vi "GetName.vi"(8 "error in (no error)":errorcluster, 11 "Konvolucio MCAN120803 Adapter Class in":refnum<class "Konvolucio MCAN120803 Adapter Class.lvclass">) -> (0 "error out":errorcluster, 2 "Value":string, 3 "Konvolucio MCAN120803 Adapter Class out":refnum<class "Konvolucio MCAN120803 Adapter Class.lvclass">)   [LabVIEW 2011, in "Konvolucio MCAN120803 Adapter Class.lvclass"]
uses:
  Konvolucio MCAN120803 Adapter Class.lvclass
  Generic CAN Adapter/GenericCanAdapterClass.lvclass
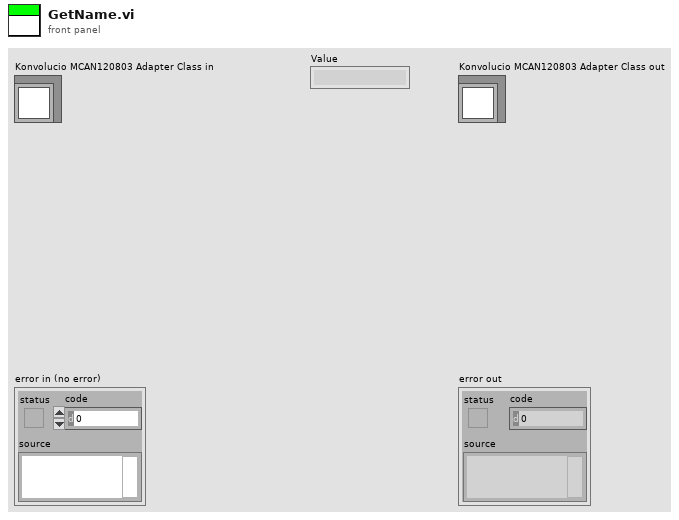
[diagram p1: front panel]
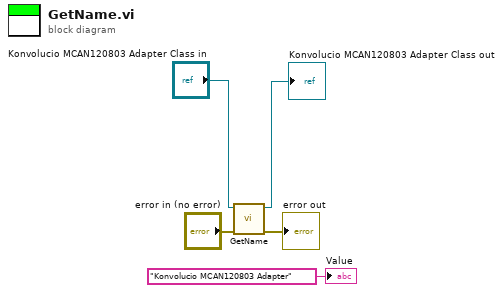
[diagram p0: block diagram]
diagram:
  n1 = call-parent "GetName.vi"("error in (no error)"="error in (no error)", "GenericCanAdapterClass in"="Konvolucio MCAN120803 Adapter Class in") -> ("error out"=→"error out":errorcluster, "GenericCanAdapterClass out"=→"Konvolucio MCAN120803 Adapter Class out":refnum<class "Konvolucio MCAN120803 Adapter Class.lvclass">)  [unwired: 7 in, 1 out]
  "Value" <- "Konvolucio MCAN120803 Adapter" ("Value")
